vi "Fit_ParabolaEM.vi"(6 "DY":ext[](array[numeric])=[1.0, 1.0, 1.0, 1.0, 1.0, 1.0] format="%.2e", 7 "Y":ext[](array[numeric])=[17.0, 6.0, 1.0, 2.0, 9.0, 22.0] format="%.2e", 9 "X":ext[](array[numeric])=[-2.0, -1.0, 0.0, 1.0, 2.0, 3.0] format="%.2e") -> (0 "Degrees of freedom":i32=3, 1 "Chi square":ext=13.257575757575757575 format="%.4e", 2 "Error Matrix":dbl[][](array[numeric])=[[0.3606060606060606, 0.03636363636363638, -0.060606060606060656], [0.036363636363636424, 0.3818181818181819, -0.13636363636363638], [-0.06060606060606063, -0.13636363636363638, 0.060606060606060615]] format="%.4e", 3 "m":ext[](array[numeric])=[1.378787878787861, -1.77272727272727, 2.621212121212123] format="%.4e")   [LabVIEW 2014]
uses:
  <vilib>/Analysis/baseanly.llb/A x Vector.vi
  <vilib>/Analysis/baseanly.llb/Real Inverse Matrix.vi
  <vilib>/Analysis/NI_AALBase.lvlib
panel:
  # "Y = m0+m1*X+m2*x^2"
  # "FS March,15 1999"
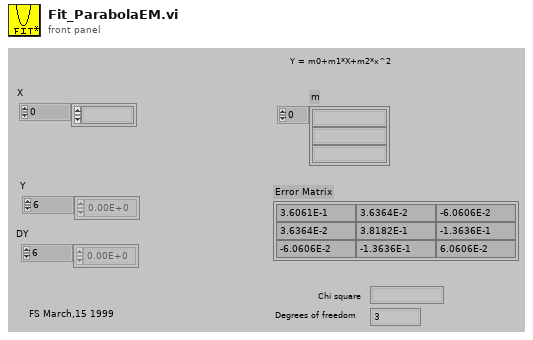
[diagram p1: front panel]
types:
  T1 = typedef "NI_Matrix.lvlib/RealMatrix.ctl" = dbl[][]
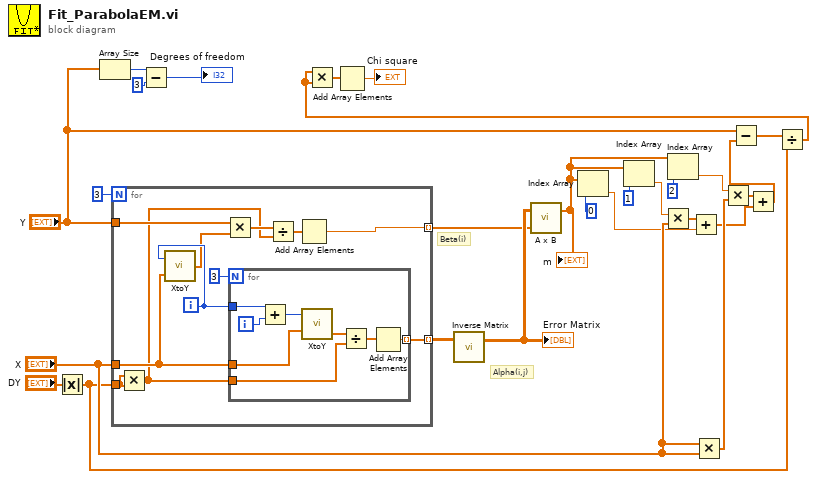
[diagram p0: block diagram]
diagram:
  # "Beta(i)"
  # "Alpha(i,j)"
  n1 = Absolute Value(x="DY") -> (abs(x)=w1:ext[])
  n2 = Array Size(array="Y") -> (size(s)=w4:i32)
  n3 = for {
    N: 3 -> [_]
    tunnel: "X" -> [w33]
    tunnel: "Y" -> [w35]
    tunnel: w1 -> [w37]
    tunnel: [w36] -> w26 mode=indexing
    tunnel: [w31] -> w24 mode=indexing
    i -> [w34]
    n4 = Multiply(x=w37, y=w37) -> (x*y=w28:ext[])
    n5 = call "XtoY.vi"("x"=w33, "y"=w34) -> ("x^y"=w32:dbl[])
    n6 = Multiply(x=w35, y=w32) -> (x*y=w29:ext[])
    n7 = for {
      N: 3 -> [_]
      tunnel: w33 -> [w43]
      tunnel: w34 -> [w46]
      tunnel: w28 -> [w41]
      tunnel: [w39] -> w36 mode=indexing
      i -> [w45]
      n8 = Add(x=w46, y=w45) -> (x+y=w44:i32)
      n9 = call "XtoY.vi"("x"=w43, "y"=w44) -> ("x^y"=w42:dbl[])
      n10 = Divide(x=w42, y=w41) -> (x/y=w40:ext[])
      n11 = Add Array Elements(numeric array=w40) -> (sum=w39:ext)
    }
    n12 = Divide(x=w29, y=w28) -> (x/y=w30:ext[])
    n13 = Add Array Elements(numeric array=w30) -> (sum=w31:ext)
  }
  n14 = Subtract(x=w4, y=3) -> (x-y=→"Degrees of freedom":i32)
  n15 = call-poly <vilib>:"Inverse Matrix.vi"("Input Matrix"=w26) -> ("Inverse Matrix"=w25:T1)  [unwired: 1 in, 1 out]
  "Error Matrix" <- w25
  n16 = call-poly <vilib>:"A x B.vi"("Vector"=w24, "A"=w25) -> ("A x Vector"=w20:dbl[])  [unwired: 1 out]
  "m" <- w20
  n17 = Index Array(array=w20, index=0) -> (element=w14:dbl)
  n18 = Index Array(array=w20, index=1) -> (element=w19:dbl)
  n19 = Multiply(x=w19, y="X") -> (x*y=w15:ext[])
  n20 = Index Array(array=w20, index=2) -> (element=w16:dbl)
  n21 = Add(x=w15, y=w14) -> (x+y=w13:ext[])
  n22 = Multiply(x="X", y="X") -> (x*y=w17:ext[])
  n23 = Multiply(x=w16, y=w17) -> (x*y=w12:ext[])
  n24 = Add(x=w12, y=w13) -> (x+y=w11:ext[])
  n25 = Subtract(x="Y", y=w11) -> (x-y=w10:ext[])
  n26 = Divide(x=w10, y=w1) -> (x/y=w8:ext[])
  n27 = Multiply(x=w8, y=w8) -> (x*y=w7:ext[])
  n28 = Add Array Elements(numeric array=w7) -> (sum=→"Chi square":ext)
